vi "Test State.vi"() -> ()   [LabVIEW 2016]
panel:
  out "number":u32
  in  "Service Affected":bool=TRUE
  in  "Warmup":bool=TRUE
  in  "Laser ON":bool=TRUE
  in  "Fault":bool=TRUE
  # "Error\n1\n3\n5\n7\n\n9\n10\n11\n\n13\n14\n15"
  # "Ready\n0\n8"
  # "Emissoin\n2"
  # "Warmup\n4\n12"
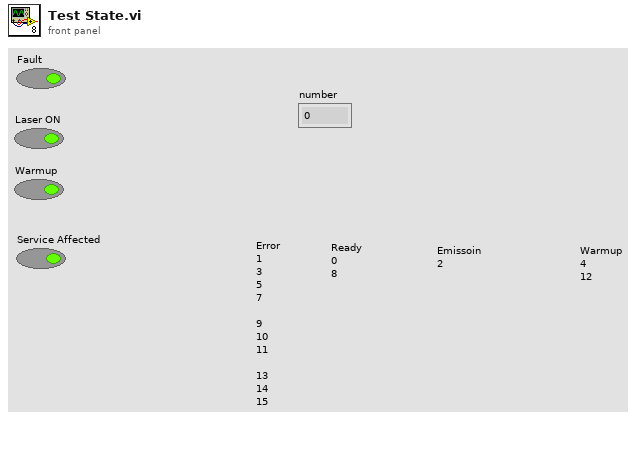
[diagram p1: front panel]
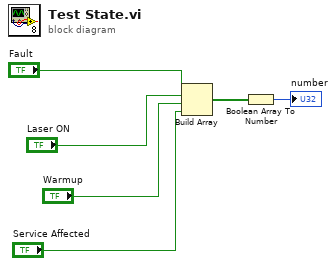
[diagram p0: block diagram]
diagram:
  n1 = Build Array("Fault", "Laser ON", "Warmup", "Service Affected") -> (w3:bool[])
  n2 = Boolean Array To Number(Boolean array=w3) -> (number=→"number":u32)
